vi "Destroy.vi"(8 "error in (no error)":errorcluster, 11 "ConfigManager in":refnum<class "ConfigManager.lvclass">) -> (0 "error out":errorcluster, 3 "ConfigManager out":refnum<class "ConfigManager.lvclass">)   [LabVIEW 2013, in "SMOConfig.lvlib" / "ConfigManager.lvclass"]
uses:
  ConfigManager.lvclass
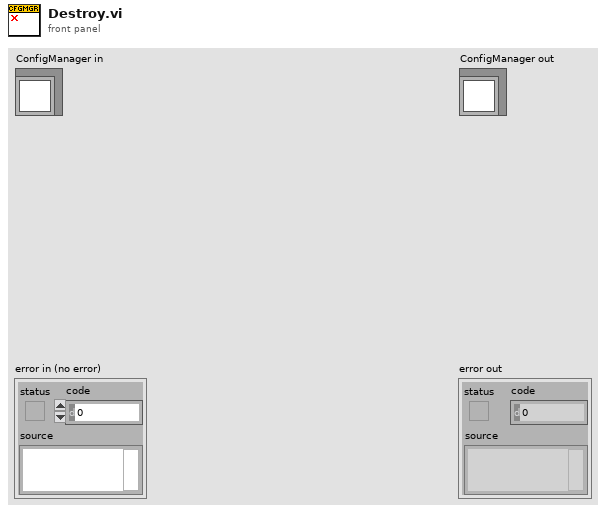
[diagram p1: front panel]
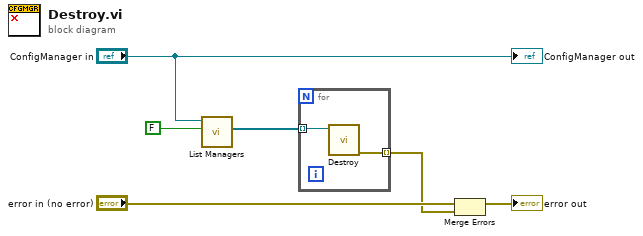
[diagram p0: block diagram]
diagram:
  n1 = call-dynamic "List Managers.vi"("Include Cache? (F)"=FALSE, "SMOConfigManager in"="ConfigManager in") -> ("List"=w3:refnum<class "ConfigManager.lvclass">[])  [unwired: 8 in, 1 out]
  n2 = for {
    tunnel: w3 -> [w8] mode=indexing
    tunnel: [w7] -> w2 mode=indexing
    n3 = call-dynamic "Destroy.vi"("ConfigManager in"=w8) -> ("error out"=w7:errorcluster)  [unwired: 9 in, 1 out]
  }
  n4 = Merge Errors("error in (no error)", w2) -> (→"error out":errorcluster)
  "ConfigManager out" <- "ConfigManager in"
